vi "make_electrode_array (SubVI).vi"(11 "Electrode settings:":T1={"DC volts (V):\n"=[0.0, 0.0, 0.0, 0.0, 0.0, 0.0, 0.0, 0.0], "Electrode to sweep:"=3, "start volt (V)"=1.5, "stop volt (V) "=1.5, "# V Steps"=1, "start freq (Hz)"=41.0, "stop freq (Hz) "=41.0, "# F steps"=1, "start DC (V)"=0.0, "stop DC (V)"=0.0, "# DC steps "=1, "Digitize electrode\ndrives?"=TRUE, "Sweep electrode?"=FALSE, "Add 0.5*V DC \noffset for amp?"=FALSE, "Use electrode \nconfig file?"=FALSE, "Path"=path "C:/GitHub/opt_lev/labview/DAQ_settings/electrode_sweep.txt", "Use arbitrary\nforce func?"=FALSE, "Voltage vs pos file"=path "C:/GitHub/opt_lev/labview/DAQ_settings/electrode_sweep.txt"}) -> (3 "Tot Electrode Arr":dbl[][](array[numeric]))   [LabVIEW 2016]
uses:
  <vilib>/Utility/file.llb/Read From Spreadsheet File (DBL).vi
panel:
  # "0"
  # "1"
  # "2"
  # "3"
  # "4"
  # "5"
  # "6"
  # "7"
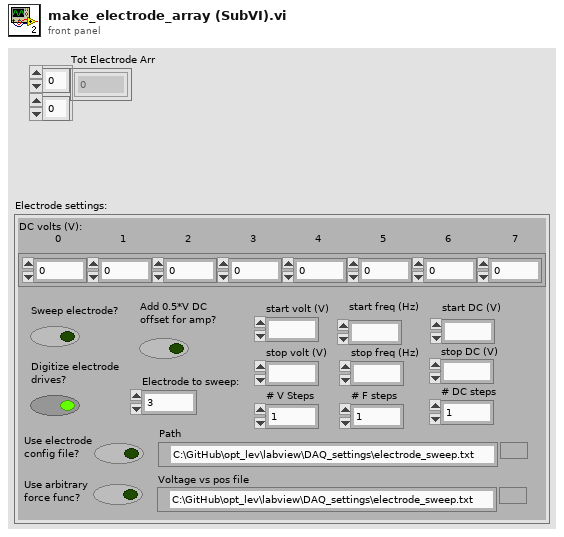
[diagram p1: front panel]
types:
  T1 = cluster{"DC volts (V):\n":dbl[], "Electrode to sweep:":i32, "start volt (V)":ext, "stop volt (V) ":ext, "# V Steps":i32, "start freq (Hz)":ext, "stop freq (Hz) ":ext, "# F steps":i32, "start DC (V)":ext, "stop DC (V)":ext, "# DC steps ":i32, "Digitize electrode\ndrives?":bool, "Sweep electrode?":bool, "Add 0.5*V DC \noffset for amp?":bool, "Use electrode \nconfig file?":bool, "Path":path, "Use arbitrary\nforce func?":bool, "Voltage vs pos file":path}
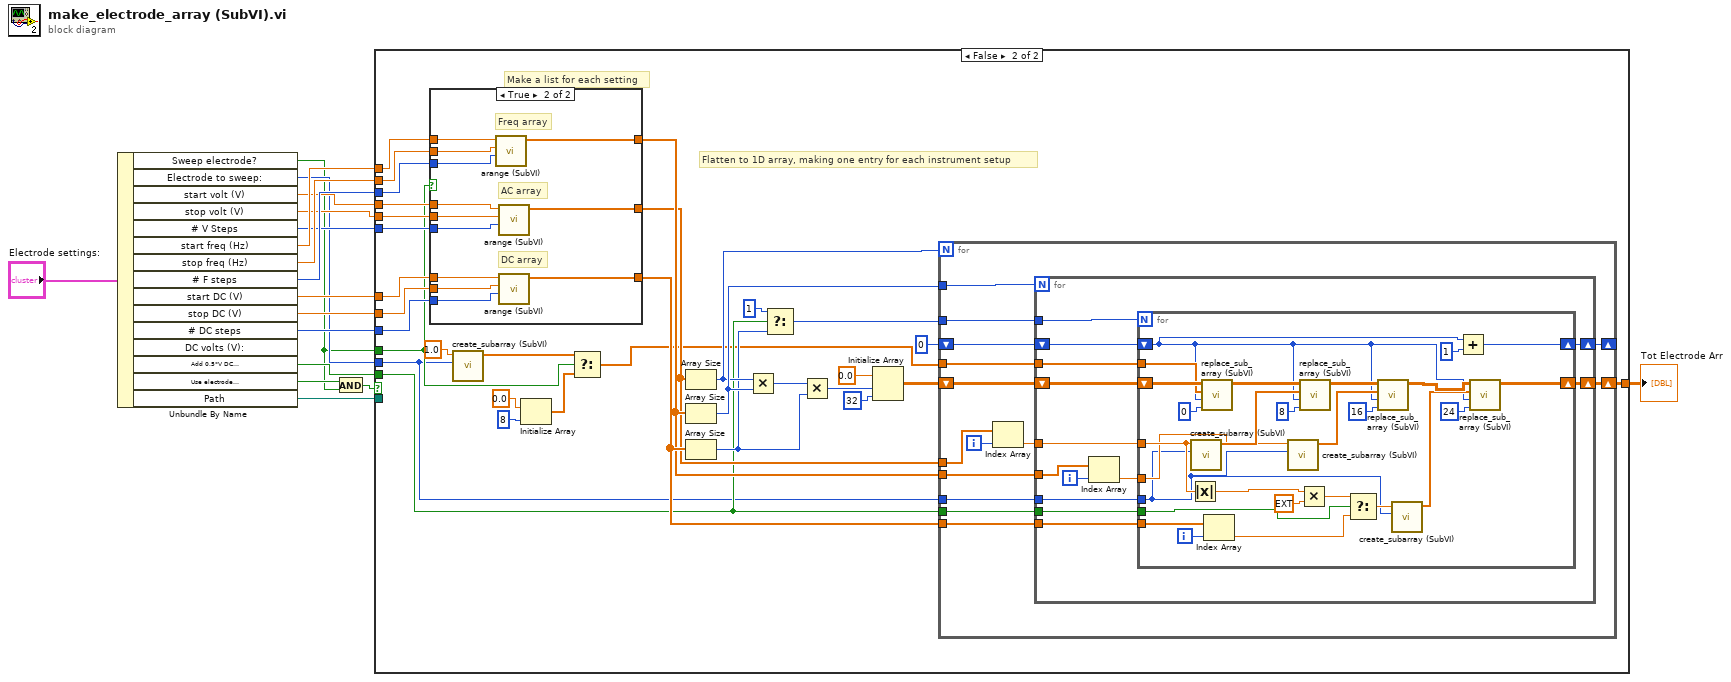
[diagram p0: block diagram]
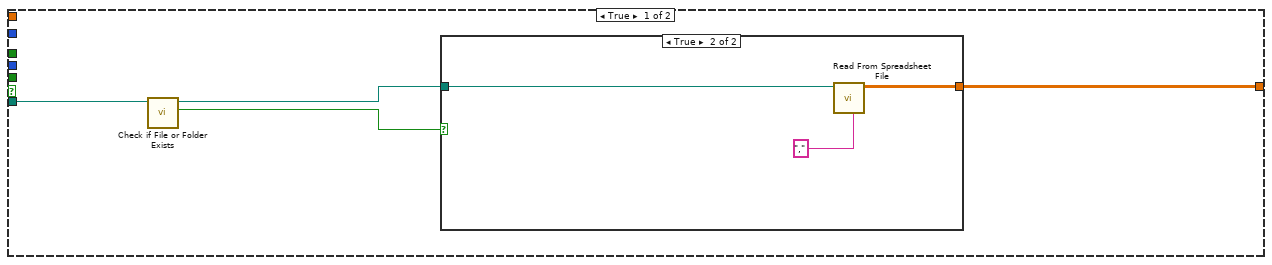
[diagram p2: hidden frame]
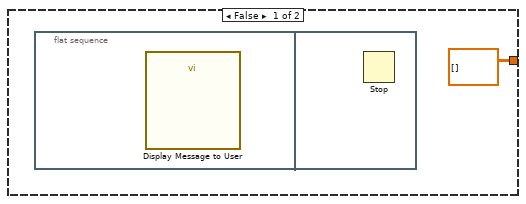
[diagram p3: hidden frame]
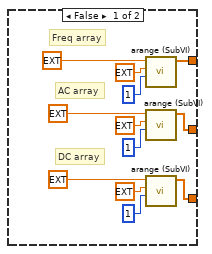
[diagram p4: hidden frame]
diagram:
  n1 = Unbundle By Name("Electrode settings:") -> ("Sweep electrode?"=w3:bool, "Electrode to sweep:"=w6:i32, "start volt (V)"=w9:ext, "stop volt (V)"=w10:ext, "# V Steps"=w11:i32, "start freq (Hz)"=w12:ext, "stop freq (Hz)"=w13:ext, "# F steps"=w14:i32, "start DC (V)"=w15:ext, "stop DC (V)"=w16:ext, "# DC steps"=w17:i32, "Add 0.5*V DC \noffset for amp?"=w7:bool, "Use electrode \nconfig file?"=w4:bool, "Path"=w5:path)  [unwired: 1 out]
  n2 = And(x=w4, y=w3) -> (x .and. y?=w2:bool)
  n3 = case shown="False" w2 {
    tunnel: w17 -> [_ w58]
    tunnel: w16 -> [_ w57]
    tunnel: w15 -> [_ w56]
    tunnel: w14 -> [_ w55]
    tunnel: w13 -> [_ w54]
    tunnel: w12 -> [_ w53]
    tunnel: w11 -> [_ w52]
    tunnel: w10 -> [_ w51]
    tunnel: w9 -> [_ w50]
    tunnel: [w18 w44] -> w8
    tunnel: w3 -> [_ w37]
    tunnel: w7 -> [_ w33]
    tunnel: w6 -> [_ w26]
    tunnel: w5 -> [w19 _]
    frame True {
      n4 = call <vilib>:"Check if File or Folder Exists.vi"("path"=w19) -> ("file or folder exists?"=w21:bool, "dup path"=w20:path)  [unwired: 8 in, 1 out]
      n5 = case shown="True" w21 {
        tunnel: w20 -> [_ w25]
        tunnel: [dbl[][] [] ("all rows") w23] -> w18
        frame False {
          n6 = flat-sequence {
            frame #0 {
              n7 = call "Display Message to User"() -> ()  [unwired: 10 in, 2 out]
            }
            frame #1 {
              n8 = Stop() -> ()  [unwired: 1 in]
            }
          }
        }
        frame True {
          n9 = call-poly <vilib>:"Read From Spreadsheet File.vi"("delimiter (\\t)"="," ("delimiter (\\t)"), "file path (dialog if empty)"=w25) -> ("all rows"=w23:dbl[][])  [unwired: 5 in, 4 out]
        }
      }
    }
    frame False {
      # "Make a list for each setting"
      # "Flatten to 1D array, making one entry for each instrument setup"
      n10 = case shown="True" w37 {
        tunnel: w50 -> [_ w136]
        tunnel: w51 -> [_ w135]
        tunnel: w52 -> [_ w134]
        tunnel: w53 -> [_ w133]
        tunnel: w54 -> [_ w132]
        tunnel: w55 -> [_ w131]
        tunnel: w56 -> [_ w130]
        tunnel: w57 -> [_ w129]
        tunnel: w58 -> [_ w128]
        tunnel: [w115 w127] -> w45
        tunnel: [w114 w126] -> w46
        tunnel: [w113 w125] -> w47
        frame False {
          # "DC array"
          # "Freq array"
          # "AC array"
          n11 = call "arange (SubVI).vi"("# Steps"=1, "stop"=ext 0.0, "start"=ext 0.0) -> ("Array"=w114:ext[])  [unwired: 8 in]
          n12 = call "arange (SubVI).vi"("# Steps"=1, "stop"=ext 0.0, "start"=ext 0.0) -> ("Array"=w115:ext[])  [unwired: 8 in]
          n13 = call "arange (SubVI).vi"("# Steps"=1, "stop"=ext 0.0, "start"=ext 0.0) -> ("Array"=w113:ext[])  [unwired: 8 in]
        }
        frame True {
          # "DC array"
          # "Freq array"
          # "AC array"
          n14 = call "arange (SubVI).vi"("# Steps"=w131, "stop"=w132, "start"=w133) -> ("Array"=w126:ext[])  [unwired: 8 in]
          n15 = call "arange (SubVI).vi"("# Steps"=w134, "stop"=w135, "start"=w136) -> ("Array"=w127:ext[])  [unwired: 8 in]
          n16 = call "arange (SubVI).vi"("# Steps"=w128, "stop"=w129, "start"=w130) -> ("Array"=w125:ext[])  [unwired: 8 in]
        }
      }
      n17 = call "create_subarray (SubVI).vi"("index"=w26, "value"=1.0) -> ("output array"=w28:dbl[])  [unwired: 9 in]
      n18 = Initialize Array(0.0 ("element"), 8 ("dimension size")) -> (w30:dbl[])
      n19 = Select(t=w28, s=w37, f=w30) -> (s? t:f=w27:dbl[])
      n20 = Array Size(array=w45) -> (size(s)=w48:i32)
      n21 = Array Size(array=w46) -> (size(s)=w49:i32)
      n22 = Array Size(array=w47) -> (size(s)=w36:i32)
      n23 = Multiply(x=w48, y=w49) -> (x*y=w39:i32)
      n24 = Select(t=1, s=w33, f=w36) -> (s? t:f=w35:i32)
      n25 = Multiply(x=w39, y=w36) -> (x*y=w40:i32)
      n26 = Initialize Array(0.0 ("element"), w40, 32 ("dimension size")) -> (w42:dbl[][])
      n27 = for {
        N: w48 -> [_]
        shift-right: [w62] -> _
        shift-left: 0 ("disabled index (row)") -> [w63]
        shift-right: [w71] -> w44
        shift-left: w42 -> [w72]
        tunnel: w45 -> [w70]
        tunnel: w46 -> [w67]
        tunnel: w47 -> [w66]
        tunnel: w49 -> [w65]
        tunnel: w35 -> [w64]
        tunnel: w27 -> [w61]
        tunnel: w33 -> [w60]
        tunnel: w26 -> [w59]
        i -> [w68]
        n28 = Index Array(array=w70, index=w68) -> (element=w69:ext)
        n29 = for {
          N: w65 -> [_]
          tunnel: w69 -> [w83]
          tunnel: w67 -> [w82]
          tunnel: w66 -> [w79]
          tunnel: w64 -> [w78]
          shift-right: [w84] -> w71
          shift-left: w72 -> [w85]
          shift-right: [w76] -> w62
          shift-left: w63 -> [w77]
          tunnel: w61 -> [w75]
          tunnel: w60 -> [w74]
          tunnel: w59 -> [w73]
          i -> [w81]
          n30 = Index Array(array=w82, index=w81) -> (element=w80:ext)
          n31 = for {
            N: w78 -> [_]
            tunnel: w83 -> [w98]
            tunnel: w80 -> [w95]
            tunnel: w79 -> [w111]
            shift-right: [w91] -> w84
            shift-left: w85 -> [w103]
            shift-right: [w104] -> w76
            shift-left: w77 -> [w86]
            tunnel: w75 -> [w102]
            tunnel: w74 -> [w108]
            tunnel: w73 -> [w87]
            i -> [w112]
            n32 = Absolute Value(x=w98) -> (abs(x)=w105:ext)
            n33 = call "create_subarray (SubVI).vi"("index"=w87, "value"=w98) -> ("output array"=w97:dbl[])  [unwired: 9 in]
            n34 = call "replace_sub_array (SubVI).vi"("Array in"=w103, "replace arr"=w102, "row"=w86, "start col"=0 ("disabled index (col)")) -> ("Array out"=w100:dbl[][])  [unwired: 5 in]
            n35 = Index Array(array=w111, index=w112) -> (element=w109:ext)
            n36 = call "create_subarray (SubVI).vi"("index"=w87, "value"=w95) -> ("output array"=w94:dbl[])  [unwired: 9 in]
            n37 = Multiply(x=w105, y=ext 1.0) -> (x*y=w107:ext)
            n38 = call "replace_sub_array (SubVI).vi"("Array in"=w100, "replace arr"=w97, "row"=w86, "start col"=8 ("disabled index (col)")) -> ("Array out"=w96:dbl[][])  [unwired: 5 in]
            n39 = Select(t=w107, s=w108, f=w109) -> (s? t:f=w89:ext)
            n40 = call "replace_sub_array (SubVI).vi"("Array in"=w96, "replace arr"=w94, "row"=w86, "start col"=16) -> ("Array out"=w92:dbl[][])  [unwired: 5 in]
            n41 = call "create_subarray (SubVI).vi"("index"=w87, "value"=w89) -> ("output array"=w88:dbl[])  [unwired: 9 in]
            n42 = Add(x=w86, y=1) -> (x+y=w104:i32)
            n43 = call "replace_sub_array (SubVI).vi"("Array in"=w92, "replace arr"=w88, "row"=w86, "start col"=24) -> ("Array out"=w91:dbl[][])  [unwired: 5 in]
          }
        }
      }
    }
  }
  "Tot Electrode Arr" <- w8
